vi "USRP Dummy_v1 (FPGA).vi"() -> ()   [LabVIEW 2016]
uses:
  <instrlib>/_niInstr/Register Bus/v1/FPGA/Public/Read Cmd Data.ctl
  <vilib>/Platform/TimedLoop/XDataNode/timing_clust.ctl
  <vilib>/Platform/TimedLoop/XDataNode/nitl_modes.ctl
  <vilib>/Platform/TimedLoop/XDataNode/wakeup.ctl
  <vilib>/rvi/Emulation/niFpgaSctlEmulationGetInTimedLoop.vi
  <vilib>/rvi/Emulation/niFpgaEmulationReportErrorSimple.vi
  <vilib>/rvi/Emulation/niFpgaGetClockAttributes.vi
  <vilib>/rvi/Emulation/niFpgaCriticalErrorInLSC.vi
  <vilib>/rvi/eio/common/nirviEmuTemplateMethod_errors.vi
  <vilib>/rvi/interface/RandomDataEmulation/niFpgaRandomDataHandleErrors.vi
  <instrlib>/_niInstr/Basic Elements/v1/FPGA/Private/Count Up U64.vi
  <vilib>/Platform/TimedLoop/XDataNode/XDataNode.xnode
  <vilib>/eio/EIONode/EIONode.xnode
  <vilib>/rvi/DataTransferAndStorage/Container/XNode/niFpgaContainer.xnode
  <vilib>/rvi/interface/RandomDataEmulation/nirviRandomDataFpgaReadWriteTemplate.vi
  <vilib>/Platform/TimedLoop/XDataNode/XDNodeRunTimeDep.lvlib
  <instrlib>/_niInstr/Register Bus/v1/FPGA/niInstr Register Bus v1 FPGA.lvlib
  <instrlib>/niUsrpRio/Config/v1/FPGA/niUsrpRio Config v1 FPGA.lvlib
  <instrlib>/_niInstr/Basic Elements/v1/FPGA/niInstr Basic Elements v1 FPGA.lvlib
panel:
  in  "Decimate (200MHz)":u32=2
  in  "Flush FIFO?":bool
  in  "Stop Transfer?":bool
  out "Min Space Available":u32
  out "Space Available":u32
  out "FPGA FIFO Depth":u32
  in  "Reset FPGA Count?":bool
  out "Send Status?":bool
  out "Samples Left to Write":u64
  in  "Number of Samples":u64
  in  "reg.host read.go rcvd 0":bool
  out "reg.notify host.go 0":bool
  in  "reg.notify host.go rcvd 0":bool
  out "reg.host read.data 0":T1
  in  "reg.reset 0":bool
  in  "RF 0/Rx/Enable":bool
  in  "RF 0/Tx/Enable":bool
  in  "RF 1/Rx/Enable":bool
  in  "RF 1/Tx/Enable":bool
  out "FPGA Count":u64
  in  "Start Transfer?":bool
  in  "Reset Timeouts?":bool
  out "Timeout Count":u64
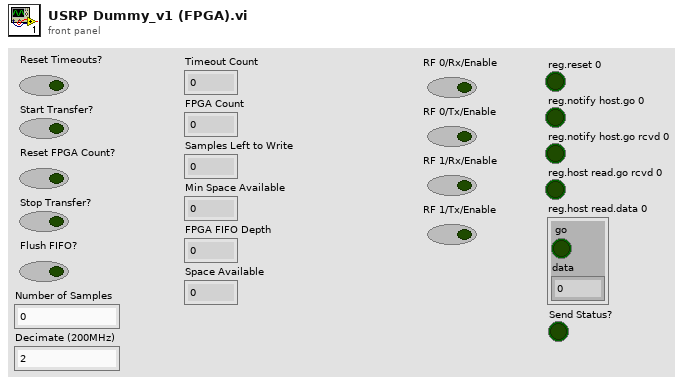
[diagram p1: front panel]
types:
  T1 = typedef "niInstr Register Bus v1 FPGA.lvlib/Read Cmd Data.ctl" = cluster{"go":bool, "data":u32}
  T2 = typedef "XDNodeRunTimeDep.lvlib/timing_clust.ctl" = cluster{"Expected End [f-1]":u64, "Actual End [f-1]":u64, "Finished Late? [f-1]":bool, "Expected End [i-1]":u64, "Actual End [i-1]":u64, "Finished Late? [i-1]":bool, "Expected Start [i]":u64, "Actual Start [i]":u64, "Expected Start [f]":u64, "Actual Start [f]":u64, "Source Name":string, "Structure Name":string, "Period":i64, "Deadline":i64, "Offset":i64, "Start":i64, "Priority":i32, "Timeout":i32, "Mode":T3, "Wakeup Reason":T4, "Error":errorcluster, "Source Type":string, "Secondary Source Type":string, "Global End Time":u64, "Global Start Time":u64, "Frame Duration":u64, "Iteration Duration":u64, "Assigned CPU":i32, "I/O Scan Engine Mode":u32}
  T3 = typedef "XDNodeRunTimeDep.lvlib/nitl_modes.ctl" = enum32{"No Change", "Process missed periods, maintain original phase", "Discard missed periods, maintain original phase", "Process missed periods, ignore original phase", "Discard missed periods, ignore original phase"}
  T4 = typedef "XDNodeRunTimeDep.lvlib/wakeup.ctl" = enum32{"Normal", "Aborted", "Asynchronous wakeup", "Timing source error", "Timed loop error", "Timeout"}
  T5 = cluster{"DAC FIFO Reset":refnum<k21>, "RF 0 Rx Swap IQ":refnum<k21>, "RF 0 Rx Negate I":refnum<k21>, "RF 0 Rx Negate Q":refnum<k21>, "RF 0 Rx Data Valid":refnum<k21>, "RF 0 Rx Data Ever Invalid":refnum<k21>, "clear RF 0 Rx Data Ever Invalid":refnum<k21>, "RF 0 Tx Swap IQ":refnum<k21>, "RF 0 Tx Negate I":refnum<k21>, "RF 0 Tx Negate Q":refnum<k21>, "RF 1 Rx Swap IQ":refnum<k21>, "RF 1 Rx Negate I":refnum<k21>, "RF 1 Rx Negate Q":refnum<k21>, "RF 1 Rx Data Valid":refnum<k21>, "RF 1 Rx Data Ever Invalid":refnum<k21>, "clear RF 1 Rx Data Ever Invalid":refnum<k21>, "RF 1 Tx Swap IQ":refnum<k21>, "RF 1 Tx Negate I":refnum<k21>, "RF 1 Tx Negate Q":refnum<k21>}
  T6 = typedef "niUsrpRio Synchronization v1 FPGA.lvlib/Resources.ctl" = cluster{"master":refnum<k21>, "meas.enable":refnum<k21>, "meas.ready":refnum<k21>, "meas.reset":refnum<k21>, "meas.arm":refnum<k21>, "meas.valid":refnum<k21>, "meas.value":refnum<k21>, "meas.oversample factor":refnum<k21>, "cptr":refnum<k21>, "cptr.adjust":refnum<k21>, "cptr.period":refnum<k21>}
  T7 = typedef "niUsrpRio Time v1 FPGA.lvlib/Time Resources.ctl" = cluster{"reset":refnum<k21>, "time":refnum<k21>, "time.previous cptr":refnum<k21>, "new time":refnum<k21>, "new time.when":refnum<k21>, "new time.set":refnum<k21>, "which edge of ref":refnum<k21>, "pps source":refnum<k21>, "internal pps period":refnum<k21>}
  T8 = typedef "niUsrpRio Time v1 FPGA.lvlib/Future Event Resources.ctl" = cluster{"reset":refnum<k21>, "future event.time":refnum<k21>, "future event.ready":refnum<k21>, "future event.set":refnum<k21>, "future event.clear":refnum<k21>, "future event.set in past":refnum<k21>}
  T9 = cluster{"time.resources":T7, "future event.resources":T8, "future event.resources":T8, "future event.resources":T8}
  T10 = typedef "niInstr Register Bus v1 FPGA.lvlib/Register Instruction.ctl" = cluster{"subsystem":u8, "address":u16, "data":u32, "valid":bool, "read":bool}
  T11 = typedef "niInstr Register Bus v1 FPGA.lvlib/Read Completion.ctl" = cluster{"data":u32, "valid":bool}
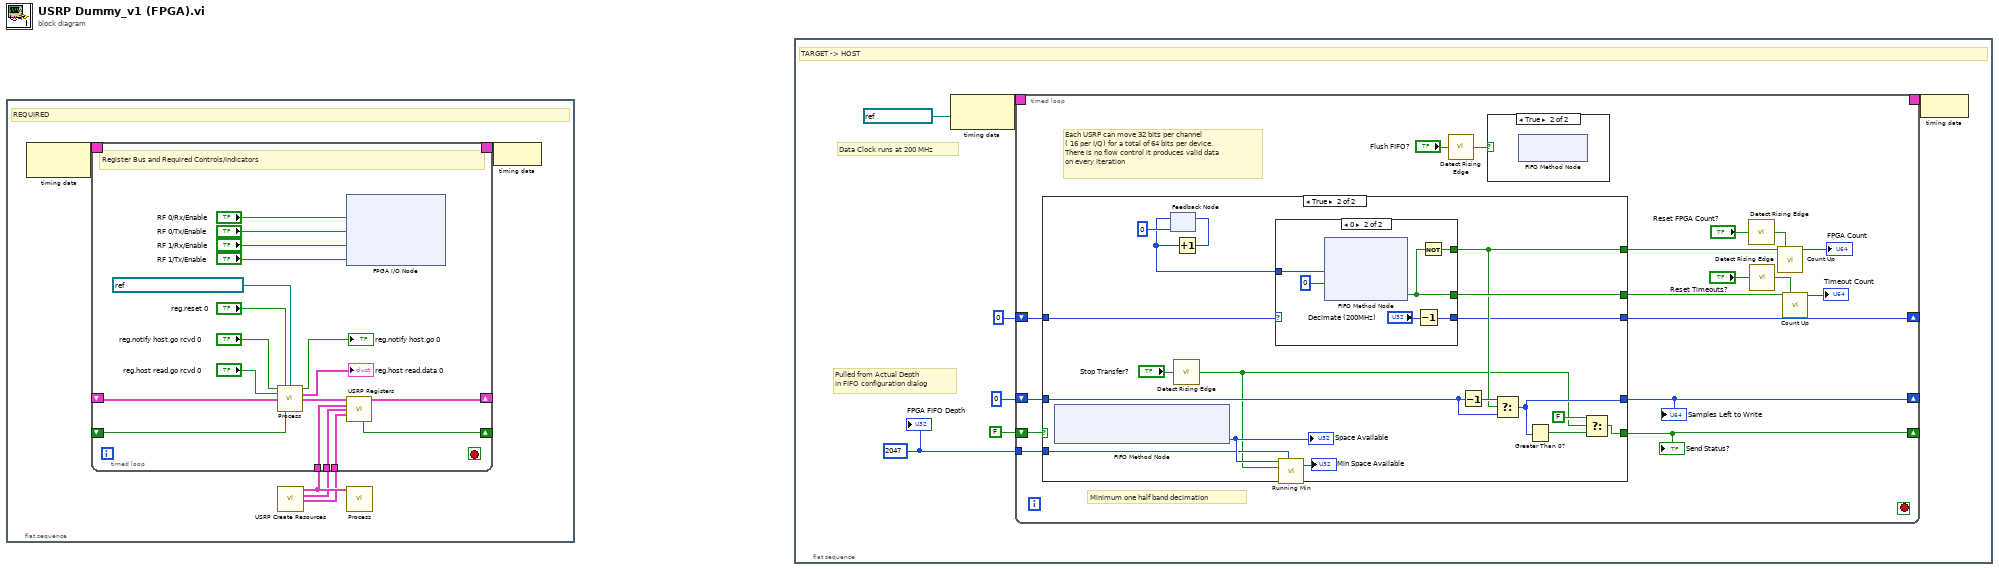
[diagram p0: block diagram]
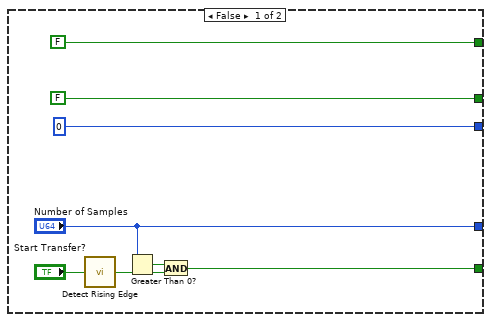
[diagram p3: hidden frame]
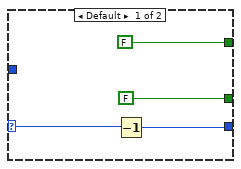
[diagram p4: hidden frame]
diagram:
  n1 = flat-sequence {
    frame #0 {
      # "REQUIRED"
      n2 = node-c288() -> (w5:T2)  [unwired: 1 in]
      n3 = call "USRP Create Resources.vi"() -> ("config.resources"=w3:T5, "sync.resources"=w2:T6, "time.resources"=w1:T9)  [unwired: 13 in]
      n4 = timed-loop "Register Bus and Required Controls/Indicators" {
        timing: w5 -> [_]
        timing-out: [_] -> w4
        shift-right: [w20] -> _
        shift-left: _ -> [w19]
        shift-right: [w14] -> _
        shift-left: _ -> [w18]
        tunnel: w3 -> [w12]
        tunnel: w2 -> [w11]
        tunnel: w1 -> [w10]
        stop <- _ stop-if-true
        # "Register Bus and Required Controls/Indicators"
        n5 = call <instrlib>:"Process.vi"("reg.notify host.go rcvd"="reg.notify host.go rcvd 0", "reg.reset"="reg.reset 0", "reg.host instruction fifo"=refnum<k21> "reg.host instruction fifo 0", "reg.host read.go rcvd"="reg.host read.go rcvd 0", "read completion"=w19, "ready for output"=w18) -> ("reg.notify host.go"=→"reg.notify host.go 0":bool, "reg.host read.data"=→"reg.host read.data 0":T1, "register instruction"=w13:T10)  [unwired: 7 in]
        n6 = xnode ("FPGA I/O Node")("RF 0/Rx/Enable"="RF 0/Rx/Enable", "RF 0/Tx/Enable"="RF 0/Tx/Enable", "RF 1/Rx/Enable"="RF 1/Rx/Enable", "RF 1/Tx/Enable"="RF 1/Tx/Enable") -> ()  [unwired: 4 in, 4 out]
        n7 = call "USRP Registers.vi"("register instruction"=w13, "config.resources"=w12, "sync.resources"=w11, "time.resources"=w10) -> ("read completion out"=w20:T11, "ready for input"=w14:bool)  [unwired: 10 in]
      }
      n8 = call <instrlib>:"Process.vi"("resources"=w3) -> ()  [unwired: 15 in]
      n9 = node-c288(w4) -> ()
    }
  }
  n10 = flat-sequence {
    frame #0 {
      w29 = u32 2047 ("FPGA FIFO Depth")
      # "Pulled from Actual Depth\nin FIFO configuration dialog"
      # "Data Clock runs at 200 MHz"
      # "TARGET -> HOST"
      n11 = node-c288(refnum<k21> "Data Clock" ("Source Name")) -> (w34:T2)
      n12 = timed-loop {
        timing: w34 -> [_]
        timing-out: [_] -> w33
        shift-right: [w51] -> _
        shift-left: FALSE ("send data?") -> [w50]
        shift-right: [w48] -> _
        shift-left: u64 0 ("samples to write") -> [w49]
        tunnel: w29 -> [w47]
        shift-right: [w40] -> _
        shift-left: u32 0 ("samples to write") -> [w39]
        stop <- _ stop-if-true
        # "Each USRP can move 32 bits per channel\n( 16 per I/Q) for a total of 64 bits per device.\nThere is no flow control it produces valid data\non every iteration"
        # "Minimum one half band decimation"
        n13 = case shown="True" w50 {
          tunnel: [FALSE ("Timed Out?") w66] -> w43
          tunnel: [FALSE ("Timed Out?") w67] -> w42
          tunnel: [w55 w68] -> w51
          tunnel: w49 -> [_ w75]
          tunnel: ["Number of Samples" w76] -> w48
          tunnel: w47 -> [_ w73]
          tunnel: [u32 0 w61] -> w40
          tunnel: w39 -> [_ w62]
          frame False {
            n14 = call <instrlib>:"Detect Rising Edge.vi"("signal"="Start Transfer?") -> ("edge detected"=w56:bool)  [unwired: 14 in]
            n15 = Greater Than 0?(x="Number of Samples") -> (x > 0?=w54:bool)
            n16 = And(x=w54, y=w56) -> (x .and. y?=w55:bool)
          }
          frame True {
            n17 = xnode ("FIFO Method Node")() -> ("Number of Elements to Write"=w74:u32)  [unwired: 1 in, 1 out]
            "Space Available" <- w74
            n18 = feedback #1(u64 0) -> (w60:u64)
            n19 = call <instrlib>:"Detect Rising Edge.vi"("signal"="Stop Transfer?") -> ("edge detected"=w63:bool)  [unwired: 14 in]
            n20 = Increment(x=w60) -> (x+1=w64:u64)
            n21 = feedback-in #1(w64) -> ()
            n22 = case shown="0" w62 {
              selector: w62 -> [w79 _]
              tunnel: w60 -> [_ w87]
              tunnel: [FALSE ("Timed Out?") w86] -> w67
              tunnel: [FALSE ("Timed Out?") w85] -> w66
              tunnel: [w78 w82] -> w61
              frame Default {
                n23 = Decrement(x=w79) -> (x-1=w78:u32)
              }
              frame 0 {
                n24 = xnode ("FIFO Method Node")("Element"=w87, "Timeout"=0) -> ("Timed Out?"=w86:bool)  [unwired: 1 in, 1 out]
                n25 = Decrement(x="Decimate (200MHz)") -> (x-1=w82:u32)
                n26 = Not(x=w86) -> (.not. x?=w85:bool)
              }
            }
            n27 = call "Running Min.vi"("Starting Min"=w73, "Reset"=w63, "Next Value"=w74) -> ("Running Min"=→"Min Space Available":u32)  [unwired: 4 in]
            n28 = Decrement(x=w75) -> (x-1=w77:u64)
            n29 = Select(t=w77, s=w66, f=w75) -> (s? t:f=w76:u64)
            n30 = Greater Than 0?(x=w76) -> (x > 0?=w69:bool)
            n31 = Select(t=FALSE, s=w63, f=w69) -> (s? t:f=w68:bool)
          }
        }
        "Samples Left to Write" <- w48
        "Send Status?" <- w51
        n32 = call <instrlib>:"Detect Rising Edge.vi"("signal"="Flush FIFO?") -> ("edge detected"=w45:bool)  [unwired: 14 in]
        n33 = case shown="True" w45 {
          frame False {
          }
          frame True {
            n34 = xnode ("FIFO Method Node")() -> ()  [unwired: 1 in, 1 out]
          }
        }
        n35 = call <instrlib>:"Detect Rising Edge.vi"("signal"="Reset FPGA Count?") -> ("edge detected"=w37:bool)  [unwired: 14 in]
        n36 = call <instrlib>:"Detect Rising Edge.vi"("signal"="Reset Timeouts?") -> ("edge detected"=w35:bool)  [unwired: 14 in]
        n37 = call-poly <instrlib>:"Count Up.vi"("increment"=w43, "reset"=w37) -> ("count out"=→"FPGA Count":u64)  [unwired: 13 in]
        n38 = call-poly <instrlib>:"Count Up.vi"("increment"=w42, "reset"=w35) -> ("count out"=→"Timeout Count":u64)  [unwired: 13 in]
      }
      n39 = node-c288(w33) -> ()
      "FPGA FIFO Depth" <- w29
    }
  }
